vi "initializeBoard.vi"(8 "error in (no error)":errorcluster, 10 "Board":i32[][](array[numeric]), 11 "SudukuState in":refnum<class "SudokuState.lvclass">) -> (0 "error out":errorcluster, 3 "SudukuState out":refnum<class "SudokuState.lvclass">)   [LabVIEW 2014, in "SudokuState.lvclass"]
uses:
  <userlib>/AdvancedDataStructures/ClassBased/Applications/SudukuSolver/SudukuState/SudokuState.lvclass
  <userlib>/AdvancedDataStructures/ClassBased/Applications/SudukuSolver/SudukuState/SudokuState.lvclass/SudokuState.ctl
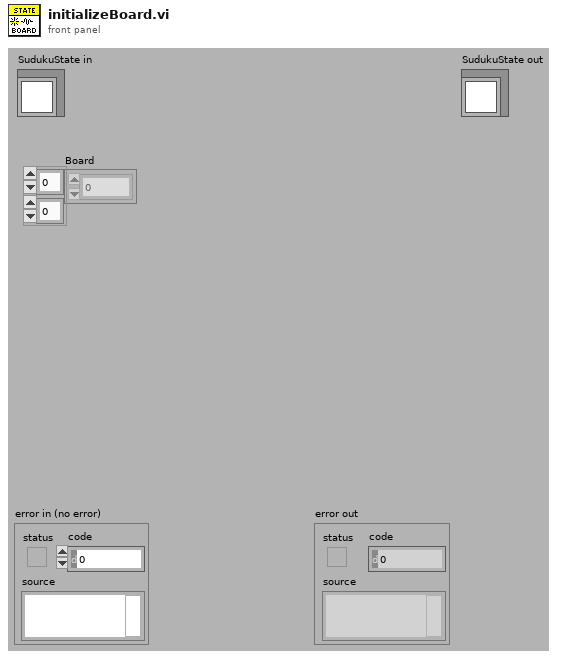
[diagram p1: front panel]
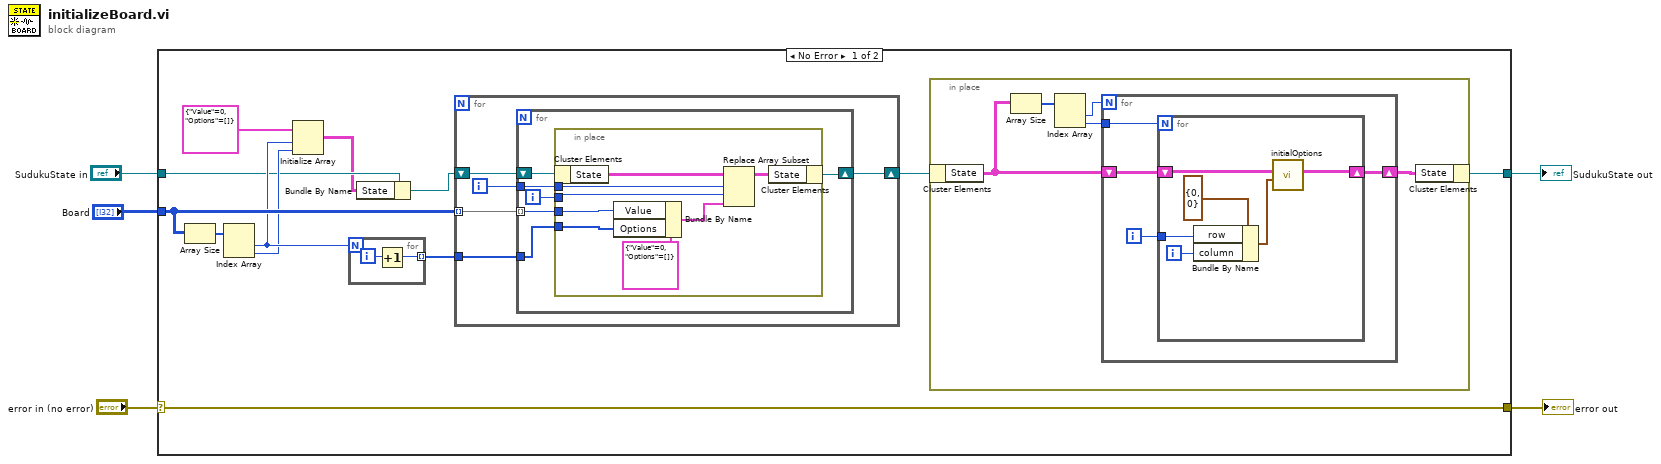
[diagram p0: block diagram]
diagram:
  n1 = case shown="No Error" "error in (no error)" {
    selector: "error in (no error)" -> [w17 w55]
    tunnel: [w17 w55] -> w4
    tunnel: [w12 w54] -> w2
    tunnel: "SudukuState in" -> [w8 w54]
    tunnel: "Board" -> [w16 _]
    frame No Error {
      n2 = Array Size(array=w16) -> (size(s)=w15:i32[])
      n3 = Index Array(array=w15) -> (element #1=w11:i32, element #2=w10:i32)  [unwired: 2 in]
      n4 = Initialize Array(cluster{"Value":i32, "Options":i32[]} {"Value"=0, "Options"=[]} ("Cell"), w11, w10) -> (w6:cluster{"Value":i32, "Options":i32[]}[][])
      n5 = for {
        N: w11 -> [_]
        tunnel: [w33] -> w14 mode=indexing
        i -> [w34]
        n6 = Increment(x=w34) -> (x+1=w33:i32)
      }
      n7 = Bundle By Name(cluster=w8, "State"=w6) -> (w7:refnum<class "SudokuState.lvclass">)
      n8 = for {
        tunnel: w16 -> [w39] mode=indexing
        shift-right: [w37] -> w13
        shift-left: w7 -> [w38]
        tunnel: w14 -> [w35]
        i -> [w36]
        n9 = for {
          tunnel: w39 -> [w41] mode=indexing
          shift-right: [w44] -> w37
          shift-left: w38 -> [w45]
          tunnel: w36 -> [w43]
          tunnel: w35 -> [w40]
          i -> [w42]
          n10 = in-place {
            in-place-border: w43 -> [w49]
            in-place-border: w42 -> [w47]
            in-place-border: w41 -> [w53]
            in-place-border: w40 -> [w52]
            n11 = in-place-cluster #1(w45) -> ("State"=w51:cluster{"Value":i32, "Options":i32[]}[][])
            n12 = Bundle By Name(cluster=cluster{"Value":i32, "Options":i32[]} {"Value"=0, "Options"=[]} ("Cell"), "Value"=w53, "Options"=w52) -> (w46:cluster{"Value":i32, "Options":i32[]})
            n13 = Replace Array Subset(array=w51, new element=w46, index (row)=w49, index (col)=w47) -> (w50:cluster{"Value":i32, "Options":i32[]}[][])
            n14 = in-place-cluster #1("State"=w50) -> (w44:refnum<class "SudokuState.lvclass">)
          }
        }
      }
      n15 = in-place {
        n16 = in-place-cluster #2(w13) -> ("State"=w22:cluster{"Value":i32, "Options":i32[]}[][])
        n17 = Array Size(array=w22) -> (size(s)=w21:i32[])
        n18 = Index Array(array=w21) -> (element #1=w20:i32, element #2=w19:i32)  [unwired: 2 in]
        n19 = for {
          N: w20 -> [_]
          shift-right: [w24] -> w18
          shift-left: w22 -> [w26]
          tunnel: w19 -> [w25]
          i -> [w23]
          n20 = for {
            N: w25 -> [_]
            shift-right: [w31] -> w24
            shift-left: w26 -> [w32]
            tunnel: w23 -> [w29]
            i -> [w28]
            n21 = Bundle By Name(cluster=cluster{"row":i32, "column":i32} {"row"=0, "column"=0} ("index"), "row"=w29, "column"=w28) -> (w27:cluster{"row":i32, "column":i32})
            n22 = call <userlib>:"initialOptions.vi"("index"=w27, "State in"=w32) -> ("State out"=w31:cluster{"Value":i32, "Options":i32[]}[][])  [unwired: 9 in]
          }
        }
        n23 = in-place-cluster #2("State"=w18) -> (w12:refnum<class "SudokuState.lvclass">)
      }
    }
    frame Error {
    }
  }
  "error out" <- w4
  "SudukuState out" <- w2
